vi "Science整体图.vi"() -> ()   [LabVIEW 2014]
panel:
  in  "Chemistry":bool
  in  "Chart":bool
  in  "Calculator":bool
  in  "Atoms":bool
  in  "Spaceship":bool
  in  "Plot":bool
  in  "Percentage":bool
  in  "Partition":bool
  in  "Molecule":bool
  in  "Maths":bool
  in  "Konquest":bool
  in  "Education":bool
  in  "Educ":bool
  in  "Division":bool
  in  "Compass":bool
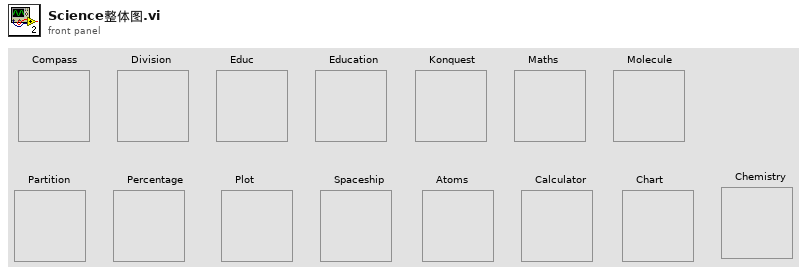
[diagram p1: front panel]
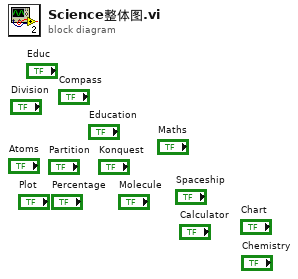
[diagram p0: block diagram]
diagram:
